vi "Render.vi"(8 "error in (no error)":errorcluster, 10 "String in":string, 11 "HorizontalRule in":refnum<class "HorizontalRule.lvclass">) -> (0 "error out":errorcluster, 2 "String out":string, 3 "HorizontalRule out":refnum<class "HorizontalRule.lvclass">)   [LabVIEW 2021, in "Markdown.lvlib" / "HorizontalRule.lvclass"]
uses:
  HorizontalRule.lvclass
  GetRuleTag.vi
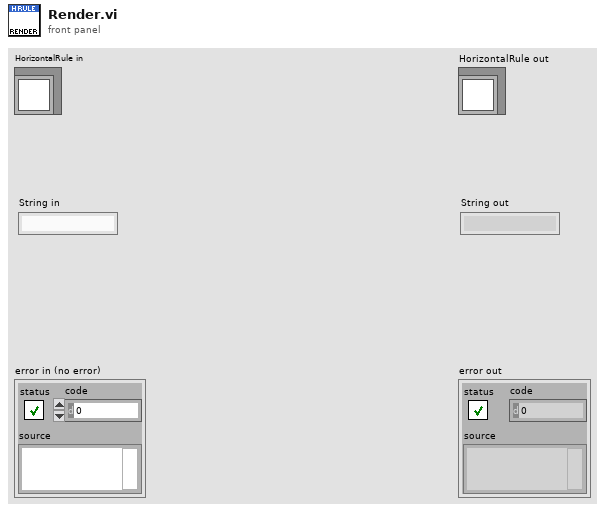
[diagram p1: front panel]
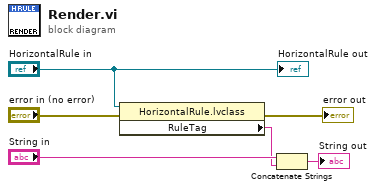
[diagram p0: block diagram]
diagram:
  n1 = property class="HorizontalRule.lvclass"(reference="HorizontalRule in", error in="error in (no error)") -> (error out=→"error out":errorcluster, "RuleTag"=w4:string)  [unwired: 1 out]
  n2 = Concatenate Strings("String in", w4) -> (→"String out":string)
  "HorizontalRule out" <- "HorizontalRule in"
